vi "NIIE_BuildCategories.vi"(7 "Main Item":string, 8 "Error":errorcluster, 9 "IconTemplates":T1[](array[typedef]), 10 "Tree":refnum<vi>, 11 "VI IE Ref":refnum<vi>) -> (0 "Error Out":errorcluster, 1 "IconTemplates Out":T1[](array[typedef]))   [LabVIEW 2021]
uses:
  MB CORE/TypeDefs/Cluster_Path&Icon.ctl
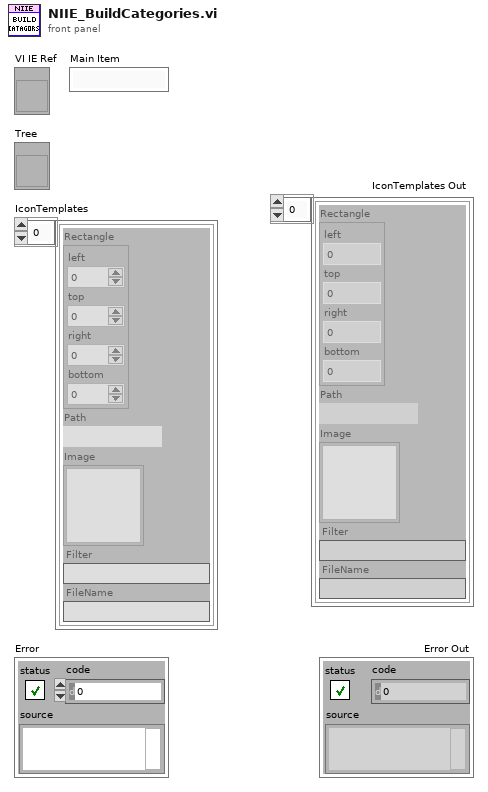
[diagram p1: front panel]
types:
  T1 = typedef "Cluster_Path&Icon.ctl" = cluster{"Rectangle":cluster{"left":i16, "top":i16, "right":i16, "bottom":i16}, "Path":path, "Image":picture, "Filter":string, "FileName":string}
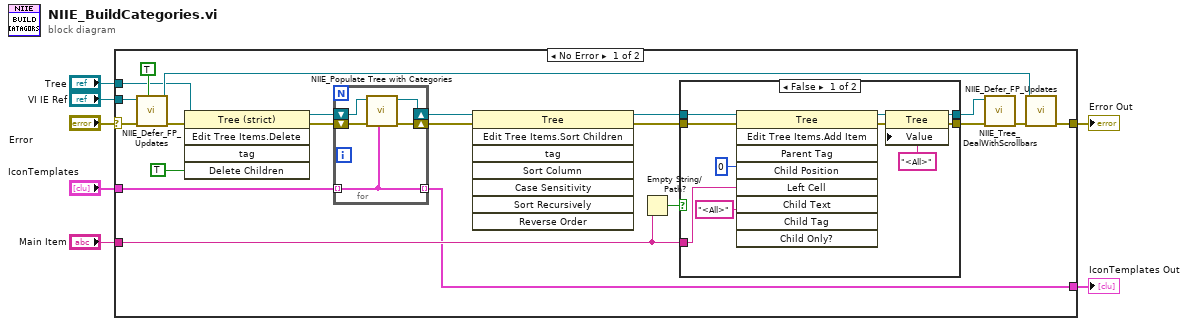
[diagram p0: block diagram]
diagram:
  n1 = case shown="No Error" "Error" {
    selector: "Error" -> [w14 w47]
    tunnel: [w17 w47] -> w6
    tunnel: "IconTemplates" -> [w28 w46]
    tunnel: "Main Item" -> [w18 _]
    tunnel: "Tree" -> [w13 _]
    tunnel: "VI IE Ref" -> [w12 _]
    tunnel: [w8 w46] -> w1
    frame No Error {
      n2 = call "NIIE_Defer_FP_Updates.vi"("Defer Panel Updates"=TRUE, "error in (no error)"=w14, "lv_icon.vi in"=w12) -> ("error out"=w16:errorcluster, "lv icon.vi out"=w15:refnum<vi>)  [unwired: 7 out]
      n3 = invoke class="Tree (strict)" method="Edit Tree Items.Delete"(reference=w13, error in=w16, "Delete Children"=TRUE ("Delete Children?")) -> (reference out=w27:refnum<vi>, error out=w26:errorcluster)  [unwired: 2 in, 3 out]
      n4 = for {
        tunnel: w28 -> [w41] mode=indexing
        shift-right: [w44] -> w22
        shift-left: w26 -> [w42]
        shift-right: [w45] -> w23
        shift-left: w27 -> [w43]
        tunnel: [w41] -> w8 mode=indexing
        n5 = call "NIIE_Populate Tree with Categories.vi"("Path & Icon"=w41, "Error"=w42, "Tree Refnum"=w43) -> ("Error Out"=w44:errorcluster, "Tree Refnum Out"=w45:refnum<vi>)  [unwired: 7 out]
      }
      n6 = invoke class="Tree" method="Edit Tree Items.Sort Children"(reference=w23, error in=w22) -> (reference out=w24:refnum<vi>, error out=w21:errorcluster)  [unwired: 6 in, 6 out]
      n7 = Empty String/Path?(string/path=w18) -> (empty?=w19:bool)
      n8 = case shown="False" w19 {
        tunnel: w18 -> [w36 _]
        tunnel: w24 -> [w35 w39]
        tunnel: w21 -> [w34 w40]
        tunnel: [w30 w40] -> w11
        tunnel: [w29 w39] -> w10
        frame False {
          n9 = invoke class="Tree" method="Edit Tree Items.Add Item"(reference=w35, error in=w34, "Child Position"=0, "Left Cell"=w36, "Child Tag"="<All>") -> (reference out=w33:refnum<vi>, error out=w32:errorcluster)  [unwired: 4 in, 7 out]
          n10 = property class="Tree"(reference=w33, error in=w32, "Value"="<All>") -> (reference out=w29:refnum<vi>, error out=w30:errorcluster)
        }
        frame True {
        }
      }
      n11 = call "NIIE_Tree_DealWithScrollbars.vi"("Error"=w11, "Tree"=w10) -> ("Error Out"=w9:errorcluster)  [unwired: 9 in]
      n12 = call "NIIE_Defer_FP_Updates.vi"("error in (no error)"=w9, "lv_icon.vi in"=w15) -> ("error out"=w17:errorcluster)  [unwired: 1 in, 8 out]
    }
    frame Error {
    }
  }
  "Error Out" <- w6
  "IconTemplates Out" <- w1
